vi "Add To Run Plan.vi"(8 "error in (no error)":errorcluster, 9 "Parameters":variant, 10 "Action":T1, 11 "AutomationContext in":refnum<class "AutomationContext.lvclass">) -> (0 "error out":errorcluster, 3 "AutomationContext out":refnum<class "AutomationContext.lvclass">)   [LabVIEW 2023, in "Automation.lvlib" / "AutomationContext.lvclass"]
uses:
  AutomationContext.lvclass
  Intent Action.ctl
  Automation Intent.ctl
  AutomationContext.lvclass/AutomationContext.ctl
  Parallel Block.ctl
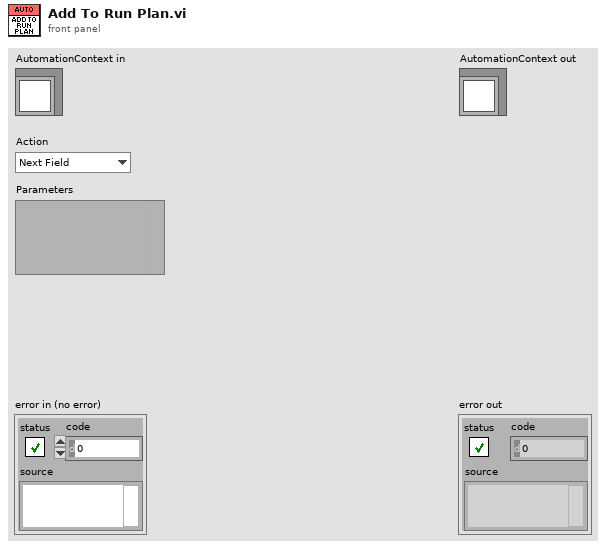
[diagram p1: front panel]
types:
  T1 = typedef "Automation.lvlib/AutomationContext.lvclass/Intent Action.ctl" = enum16{"Next Field", "Next Lane", "Set Power", "Reset Power", "Autofocus", "Start Streaming", "Delay", "Finish Run", "Open Shutter", "Close Shutter"}
  T2 = typedef "Automation.lvlib/AutomationContext.lvclass/Parallel Block.ctl" = cluster{"Tasks":T3[]}
  T3 = typedef "Automation.lvlib/AutomationContext.lvclass/Automation Intent.ctl" = cluster{"Action":T1, "Parameters":variant, "Correlation ID":u32}
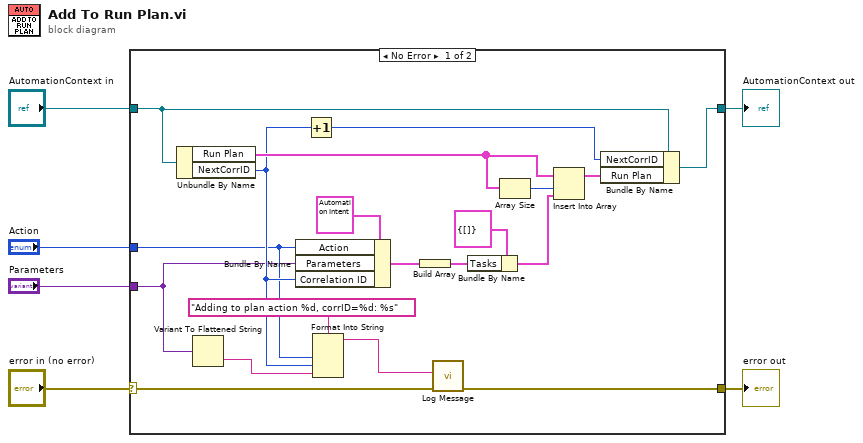
[diagram p0: block diagram]
diagram:
  n1 = case shown="No Error" "error in (no error)" {
    selector: "error in (no error)" -> [w18 w27]
    tunnel: [w17 w27] -> w5
    tunnel: [w24 w26] -> w3
    tunnel: "AutomationContext in" -> [w20 w26]
    tunnel: "Action" -> [w13 _]
    tunnel: "Parameters" -> [w12 _]
    frame No Error {
      n2 = Unbundle By Name(w20) -> ("Run Plan"=w22:T2[], "NextCorrID"=w14:u32)
      n3 = Variant To Flattened String(Variant=w12) -> (data string=w11:string)  [unwired: 1 out]
      n4 = Bundle By Name(cluster=T3 {"Action"=enum."Next Field", "Parameters"=variant, "Correlation ID"=0} ("Automation Step"), "Action"=w13, "Parameters"=w12, "Correlation ID"=w14) -> (w10:T3)
      n5 = Increment(x=w14) -> (x+1=w19:u32)
      n6 = Format Into String(format string="Adding to plan action %d, corrID=%d: %s", w13, w14, w11) -> (resulting string=w16:string)  [unwired: 2 in, 1 out]
      n7 = Build Array(w10) -> (w9:T3[])
      n8 = call "Log Message.vi"("error constant"=w18, "input"=w16) -> ("error constant 2"=w17:errorcluster)  [unwired: 8 in, 1 out]
      n9 = Bundle By Name(cluster=T2 {"Tasks"=[]} ("Parallel Block"), "Tasks"=w9) -> (w7:T2)
      n10 = Array Size(array=w22) -> (size(s)=w21:i32)
      n11 = Insert Into Array(array=w22, index=w21, new element=w7) -> (w23:T2[])
      n12 = Bundle By Name(cluster=w20, "NextCorrID"=w19, "Run Plan"=w23) -> (w24:refnum<class "AutomationContext.lvclass">)
    }
    frame Error {
    }
  }
  "error out" <- w5
  "AutomationContext out" <- w3
